vi "Puff_release3_chs.vi"() -> (5 "Plug in titles":string[](array[string]), 7 "Plug in values":string[](array[string]))   [LabVIEW 2010]
uses:
  Controls/Post_Process.ctl
  Globals/Plug_in_data_global.vi
  Globals/Meas_global.vi
  Globals/Constants_global.vi
  Globals/Dynamic_call_global.ph.vi
  <vilib>/Analysis/NI_AALPro.lvlib
panel:
  in  "Per Block Mode":T1(ring)
  in  "Averaging Samples":i32=1 min=1
  out "Valve to monitor delay (s)":dbl format="%.2f"
  out "Monitor trigger Index":dbl format="%.2f"
  out "Valve Trigger Index":dbl format="%.2f"
  out "Monitor FID":cluster{dbl, dbl, dbl[]}(graph)
  out "delay":dbl format="%.2f"
  out "Pulse Width":dbl format="%.2f"
  out "falltime":dbl format="%.2f"
  out "top":dbl format="%.2f"
  out "risetime":dbl format="%.2f"
  in  "Save Time pdf?":bool
  out "Pdf":cluster{"Axis":dbl[], dbl[]}(graph)
  in  "Histogram Time":dbl format="%.2f"
  out "Current Block No":i32
  in  "Save averaged traces?":bool
  in  "Pause Mode":T2(ring)
  in  "OK":bool
  out "No of Valid Blocks":dbl
  out "Valve Trace":dbl[](graph)
  out "FFID Trace":cluster{dbl, dbl, dbl[]}(graph)
  out "Source On":i32
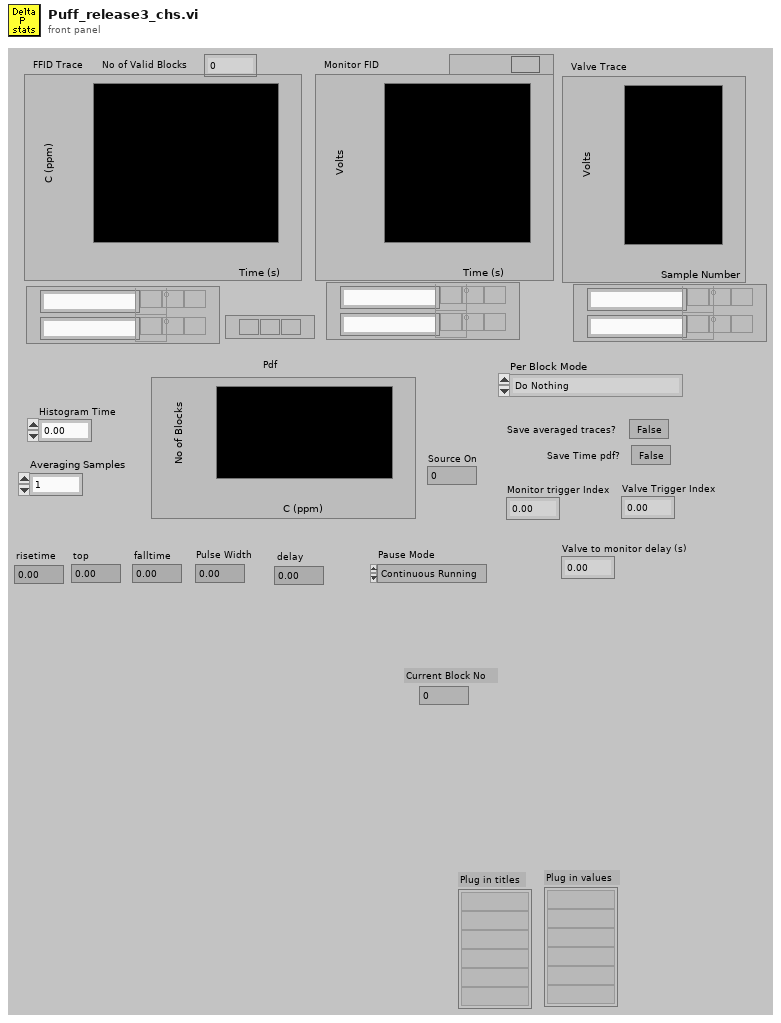
[diagram p1: front panel]
types:
  T1 = enum16{"Do Nothing", "Save Block Time Traces", "Save Jpeg plots"}
  T2 = enum16{"Continuous Running", "After Each  Block"}
  T3 = typedef "Post_Process.ctl" = enum16{"Take New Data", "Post Process Raw Data File"}
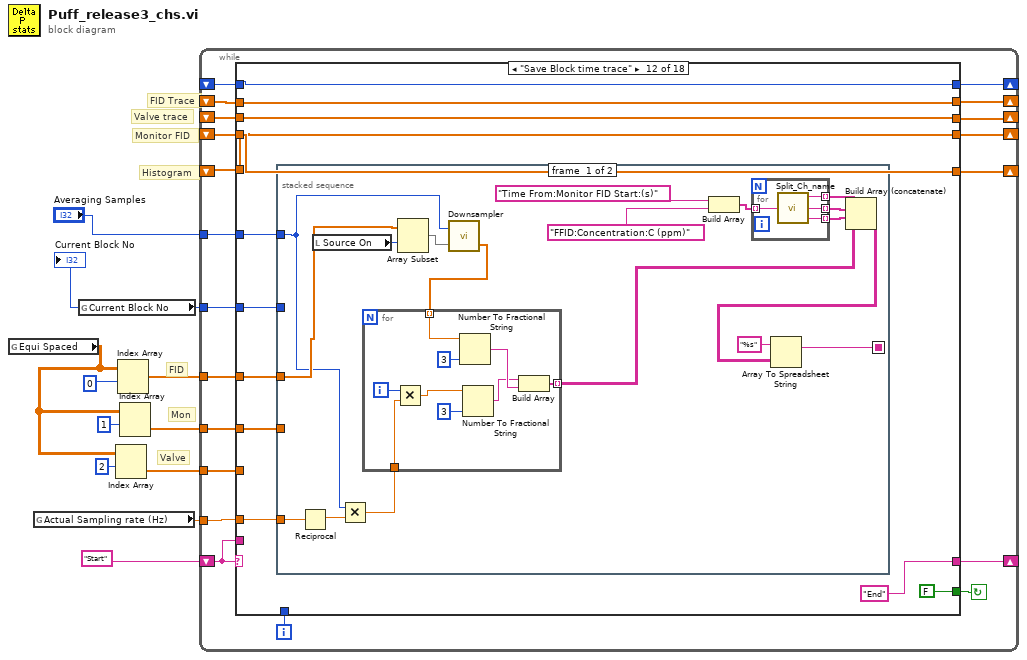
[diagram p0: block diagram]
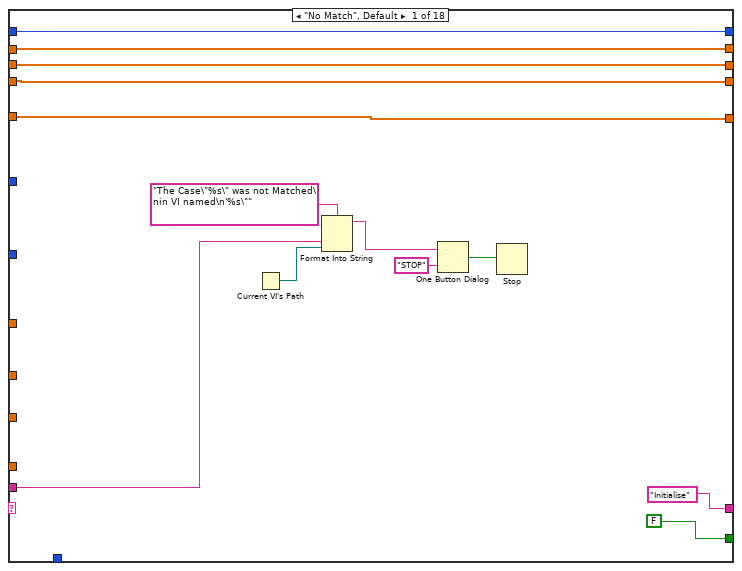
[diagram p2: hidden frame]
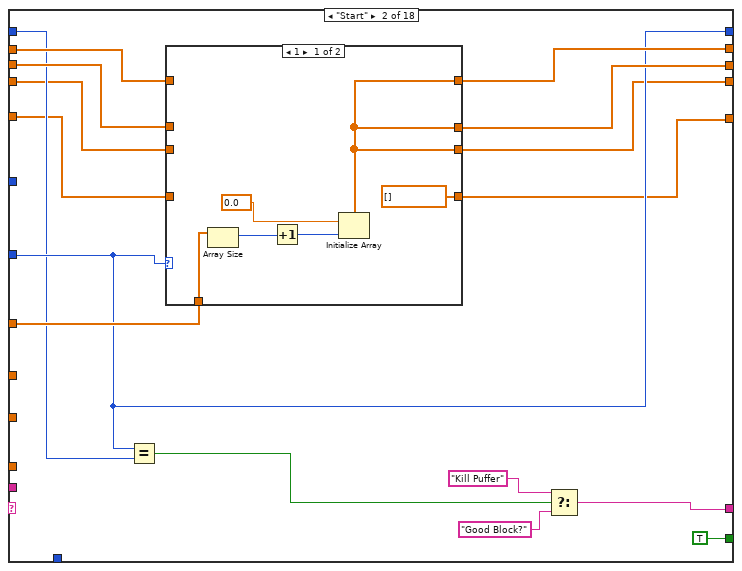
[diagram p3: hidden frame]
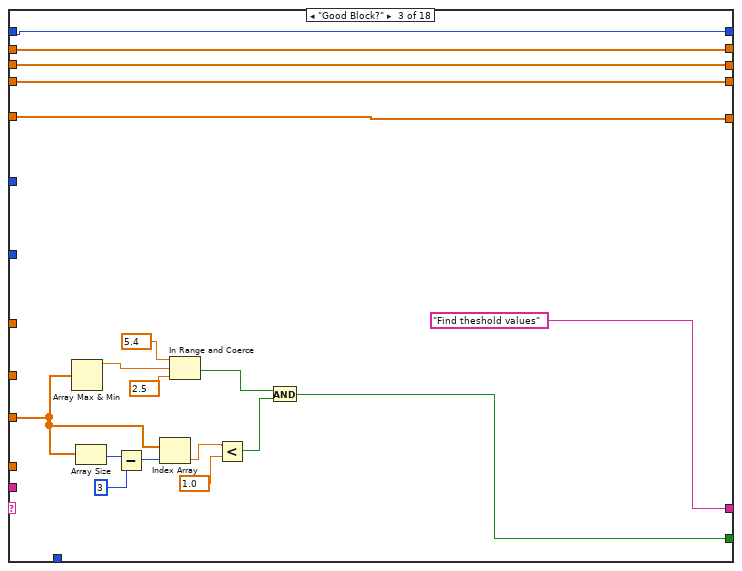
[diagram p5: hidden frame]
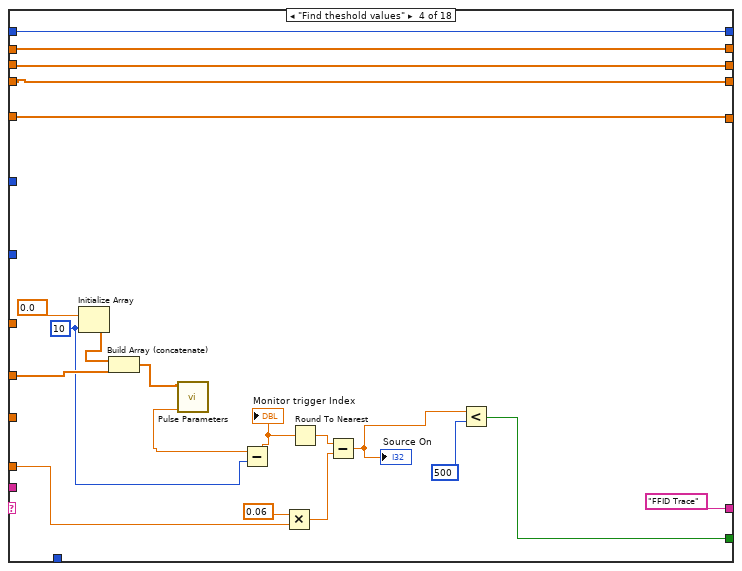
[diagram p6: hidden frame]
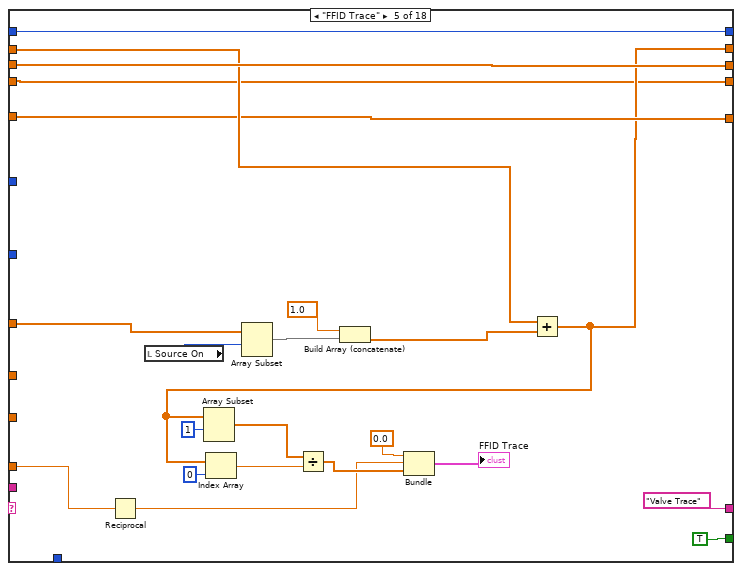
[diagram p7: hidden frame]
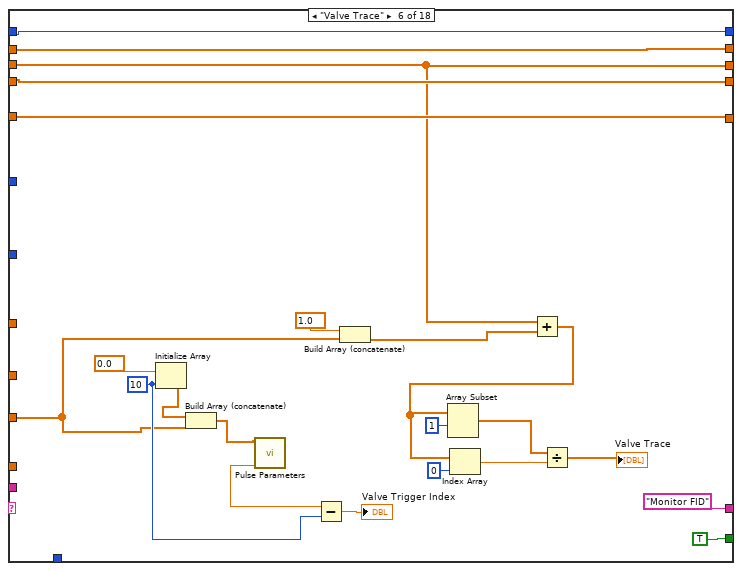
[diagram p8: hidden frame]
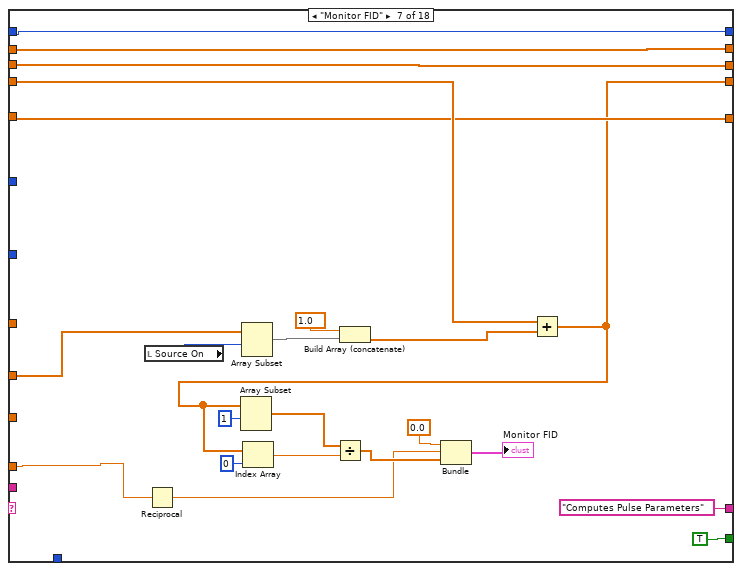
[diagram p9: hidden frame]
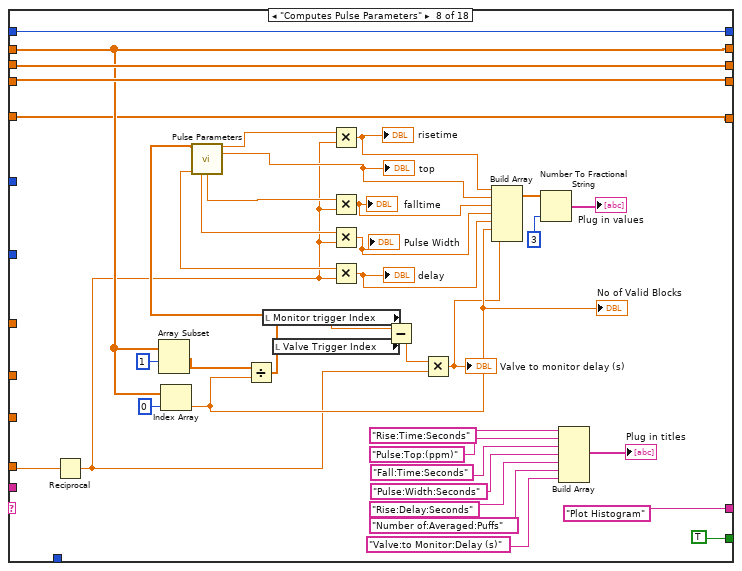
[diagram p10: hidden frame]
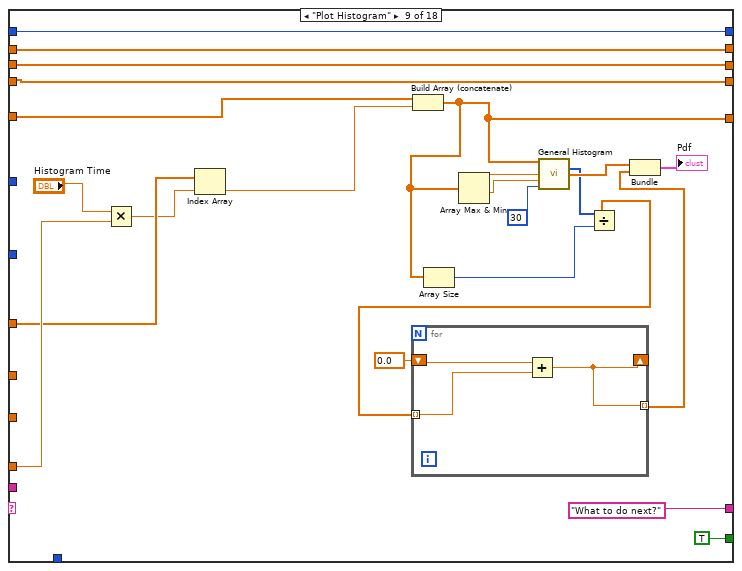
[diagram p11: hidden frame]
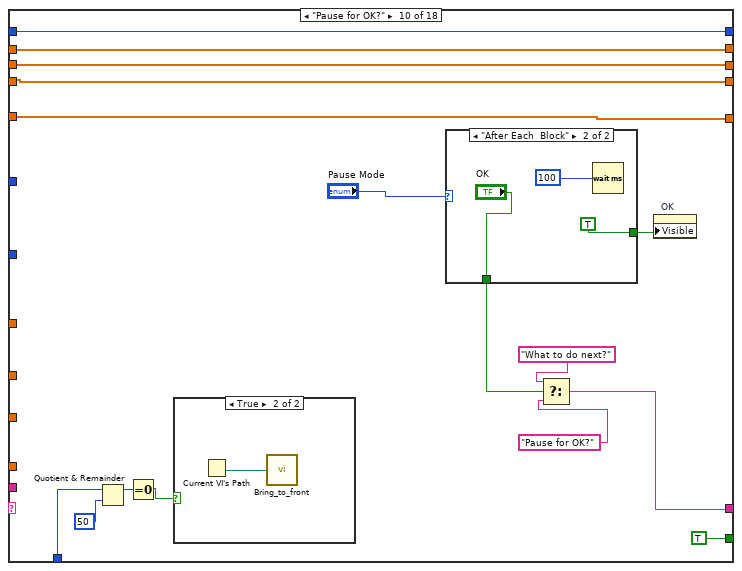
[diagram p12: hidden frame]
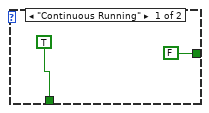
[diagram p14: hidden frame]
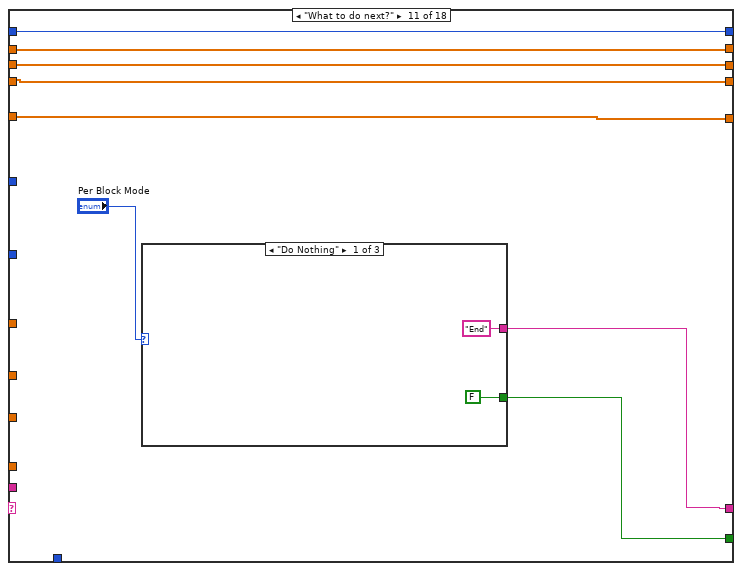
[diagram p15: hidden frame]
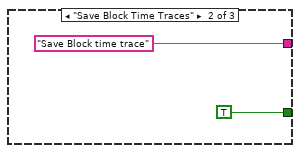
[diagram p16: hidden frame]
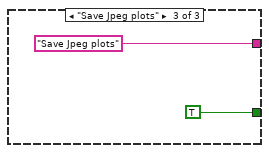
[diagram p17: hidden frame]
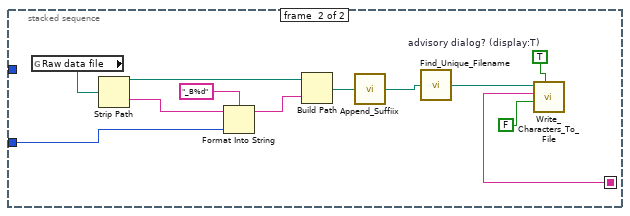
[diagram p18: hidden frame]
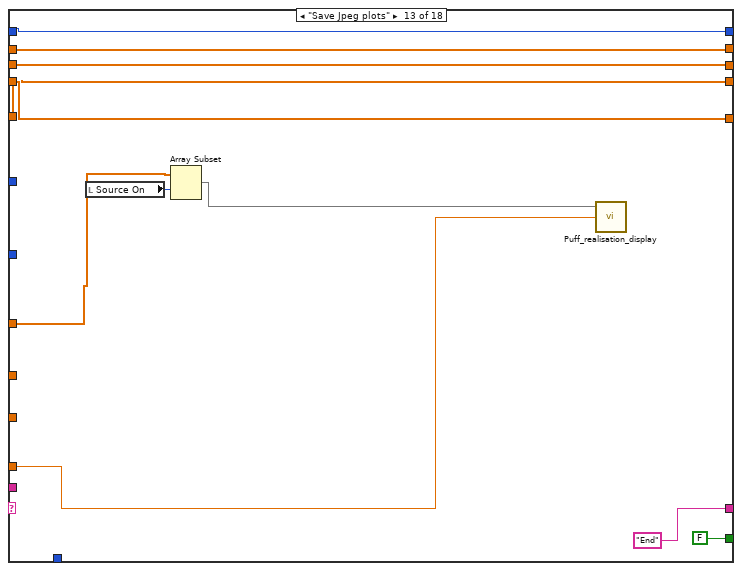
[diagram p19: hidden frame]
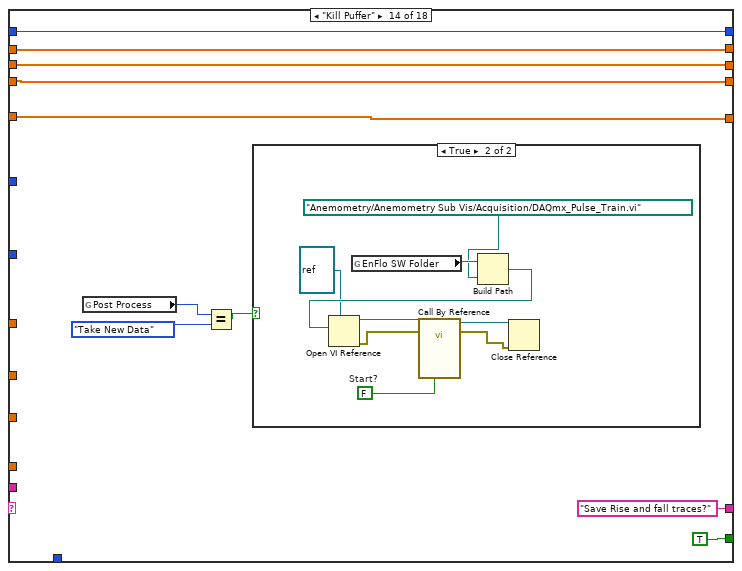
[diagram p20: hidden frame]
diagram:
  # "Valve"
  # "Mon"
  # "FID"
  # "Histogram"
  # "Monitor FID"
  # "Valve trace"
  # "FID Trace"
  n1 = global read "Plug_in_data_global.vi" "Equi Spaced"() -> (w4:dbl[][])
  n2 = global read "Meas_global.vi" "Actual Sampling rate (Hz)"() -> (w8:dbl)
  n3 = global read "Meas_global.vi" "Current Block No"() -> (w7:i32)
  "Current Block No" <- w7
  n4 = Index Array(array=w4, index (row)=2) -> (element=w3:dbl[])  [unwired: 1 in]
  n5 = Index Array(array=w4, index (row)=0) -> (element=w9:dbl[])  [unwired: 1 in]
  n6 = Index Array(array=w4, index (row)=1) -> (element=w10:dbl[])  [unwired: 1 in]
  n7 = while {
    shift-left: "Start" -> [w29]
    shift-right: [w30] -> _
    shift-right: [w28] -> _
    shift-left: _ -> [w25]
    shift-right: [w27] -> _
    shift-left: _ -> [w26]
    tunnel: w10 -> [w24]
    tunnel: w9 -> [w23]
    tunnel: w8 -> [w22]
    tunnel: w7 -> [w21]
    shift-right: [w18] -> _
    shift-left: _ -> [w19]
    shift-right: [w16] -> _
    shift-left: _ -> [w17]
    shift-right: [w14] -> _
    shift-left: _ -> [w13]
    tunnel: w3 -> [w15]
    tunnel: "Averaging Samples" -> [w12]
    i -> [w20]
    stop <- w31 continue-if-true
    n8 = case shown="\"Save Block time trace\"" w29 {
      tunnel: [FALSE TRUE ("Processing last block?") w78 w104 TRUE ("Processing last block?") TRUE ("Processing last block?") TRUE ("Processing last block?") TRUE ("Processing last block?") TRUE ("Processing last block?") TRUE ("Processing last block?") w261 FALSE ("Processing last block?") FALSE ("Processing last block?") TRUE ("Processing last block?") w360 TRUE ("Processing last block?") "Save Time pdf?" FALSE ("Processing last block?")] -> w31
      tunnel: ["Initialise" w50 "Find theshold values" "FFID Trace" "Valve Trace" "Monitor FID" "Computes Pulse Parameters" "Plot Histogram" ("f") "What to do next?" ("f") w241 w262 "End" "End" "Save Rise and fall traces?" w363 "Save Time pdf?" "Save Time pdf" "End"] -> w30
      tunnel: w29 -> [w39 _ _ _ _ _ _ _ _ _ _ _ _ _ _ _ _ _]
      tunnel: [w36 w59 w88 w107 w115 w149 w169 w182 w235 w254 w268 w286 w340 w350 w369 w376 w445 w455] -> w28
      tunnel: [w35 w57 w87 w106 w128 w131 w166 w210 w234 w253 w267 w285 w339 w349 w368 w375 w444 w454] -> w27
      tunnel: w26 -> [w35 w56 w87 w106 w128 w131 w166 w210 w234 w253 w267 w285 w339 w349 w368 w375 w444 w454]
      tunnel: w25 -> [w36 w58 w88 w107 w126 w149 w169 w182 w235 w254 w268 w286 w340 w350 w369 w376 w445 w455]
      tunnel: w24 -> [_ _ _ w100 _ _ w153 _ _ _ _ w282 _ _ _ _ _ w451]
      tunnel: w23 -> [_ w55 _ _ w127 _ _ _ w230 _ _ w281 w333 _ _ _ _ w450]
      tunnel: w22 -> [_ _ _ w94 w112 _ w154 w208 w231 _ _ w275 w330 _ _ _ _ _]
      tunnel: w21 -> [_ w54 _ _ _ _ _ _ _ _ _ w280 _ _ _ _ _ w449]
      tunnel: w20 -> [_ _ _ _ _ _ _ _ _ w251 _ _ _ _ _ _ _ _]
      tunnel: w19 -> [w34 w53 w79 w103 w121 w148 w168 w206 w233 w247 w266 w279 w336 w346 _ w372 _ w448]
      tunnel: [w34 w54 w79 w103 w121 w148 w168 w206 w233 w247 w266 w279 w336 w346 0 w372 0 w448] -> w18
      tunnel: w17 -> [w33 w47 w77 w96 w120 w141 w164 w181 w227 w246 w265 w278 w335 w342 w361 w371 w440 w446]
      tunnel: [w33 w48 w77 w96 w120 w141 w164 w181 w219 w246 w265 w278 w335 w342 w361 w371 w440 w446] -> w16
      tunnel: w15 -> [_ _ w73 _ _ w134 _ _ _ _ _ _ _ _ _ _ _ _]
      tunnel: [w32 w46 w74 w97 w109 w142 w155 w186 w216 w245 w264 w277 w334 w341 w362 w370 w439 w447] -> w14
      tunnel: w13 -> [w32 w45 w74 w97 w109 w142 w165 w186 w216 w245 w264 w277 w334 w341 w362 w370 w439 w447]
      tunnel: w12 -> [_ _ _ _ _ _ _ _ _ _ _ w276 _ _ _ _ _ _]
      frame "No Match", Default {
        n9 = Current VI's Path() -> (path=w38:path)
        n10 = Format Into String(format string="The Case\"%s\" was not Matched\nin VI named\n'%s\"" ("Format String"), w39, w38) -> (resulting string=w42:string)  [unwired: 2 in, 1 out]
        n11 = One Button Dialog(message=w42, button name ("OK")="STOP") -> (true=w40:bool)
        n12 = Stop(stop? (T)=w40) -> ()
      }
      frame "Start" {
        n13 = Equal?(x=w54, y=w53) -> (x = y?=w52:bool)
        n14 = case shown="1" w54 {
          tunnel: [w62 w70] -> w59
          tunnel: w58 -> [_ w70]
          tunnel: [w62 w69] -> w57
          tunnel: w56 -> [_ w69]
          tunnel: w55 -> [w66 _]
          tunnel: [dbl[] [] w68] -> w48
          tunnel: w47 -> [_ w68]
          tunnel: [w62 w67] -> w46
          tunnel: w45 -> [_ w67]
          frame 1 {
            n15 = Array Size(array=w66) -> (size(s)=w65:i32)
            n16 = Increment(x=w65) -> (x+1=w61:i32)
            n17 = Initialize Array(0.0 ("element"), w61) -> (w62:dbl[])
          }
          frame 2, Default {
          }
        }
        n18 = Select(t="Kill Puffer", s=w52, f="Good Block?") -> (s? t:f=w50:string)
      }
      frame "Good Block?" {
        n19 = Array Max & Min(array=w73) -> (max value=w76:dbl)  [unwired: 3 out]
        n20 = Array Size(array=w73) -> (size(s)=w72:i32)
        n21 = Subtract(x=w72, y=3) -> (x-y=w84:i32)
        n22 = Index Array(array=w73, index=w84) -> (element=w83:dbl)
        n23 = In Range and Coerce(upper limit=5.4, x=w76, lower limit=2.5 ("y")) -> (In Range?=w80:bool)  [unwired: 1 out]
        n24 = Less?(x=w83, y=1.0) -> (x < y?=w81:bool)
        n25 = And(x=w80, y=w81) -> (x .and. y?=w78:bool)
      }
      frame "Find theshold values" {
        w98 = 10 ("dimension size")
        n26 = Initialize Array(0.0, w98) -> (w99:dbl[])
        n27 = Build Array (concatenate)(w99, w100) -> (w101:dbl[])
        n28 = call <vilib>:"Pulse Parameters.vi"("X"=w101) -> ("delay"=w93:dbl)  [unwired: 14 out]
        n29 = Subtract(x=w93, y=w98) -> (x-y=w92:dbl)
        "Monitor trigger Index" <- w92
        n30 = Multiply(x=0.06 ("y"), y=w94) -> (x*y=w90:dbl)
        n31 = Round To Nearest(number=w92) -> (nearest integer value=w91:dbl)
        n32 = Subtract(x=w91, y=w90) -> (x-y=w89:dbl)
        "Source On" <- w89
        n33 = Less?(x=w89, y=500) -> (x < y?=w104:bool)
      }
      frame "FFID Trace" {
        n34 = Reciprocal(x=w112) -> (1/x=w111:dbl)
        n35 = local read "Source On"() -> (w123:i32)
        n36 = Array Subset(array=w127, index=w123) -> (w122:dbl[])  [unwired: 1 in]
        n37 = Build Array (concatenate)(1.0, w122) -> (w124:dbl[])
        n38 = Add(x=w126, y=w124) -> (x+y=w115:dbl[])
        n39 = Array Subset(array=w115, index=1) -> (w114:dbl[])  [unwired: 1 in]
        n40 = Index Array(array=w115, index=0) -> (element=w113:dbl)
        n41 = Divide(x=w114, y=w113) -> (x/y=w119:dbl[])
        n42 = Bundle(0.0, w111, w119) -> (→"FFID Trace":cluster{dbl, dbl, dbl[]})  [unwired: 1 out]
      }
      frame "Valve Trace" {
        w135 = 10 ("dimension size")
        n43 = Initialize Array(0.0, w135) -> (w136:dbl[])
        n44 = Build Array (concatenate)(w136, w134) -> (w137:dbl[])
        n45 = call <vilib>:"Pulse Parameters.vi"("X"=w137) -> ("delay"=w132:dbl)  [unwired: 14 out]
        n46 = Subtract(x=w132, y=w135) -> (x-y=→"Valve Trigger Index":dbl)
        n47 = Build Array (concatenate)(1.0, w134) -> (w150:dbl[])
        n48 = Add(x=w131, y=w150) -> (x+y=w139:dbl[])
        n49 = Array Subset(array=w139, index=1) -> (w144:dbl[])  [unwired: 1 in]
        n50 = Index Array(array=w139, index=0) -> (element=w143:dbl)
        n51 = Divide(x=w144, y=w143) -> (x/y=→"Valve Trace":dbl[])
      }
      frame "Monitor FID" {
        n52 = local read "Source On"() -> (w171:i32)
        n53 = Reciprocal(x=w154) -> (1/x=w157:dbl)
        n54 = Array Subset(array=w153, index=w171) -> (w170:dbl[])  [unwired: 1 in]
        n55 = Build Array (concatenate)(1.0, w170) -> (w172:dbl[])
        n56 = Add(x=w165, y=w172) -> (x+y=w155:dbl[])
        n57 = Array Subset(array=w155, index=1) -> (w159:dbl[])  [unwired: 1 in]
        n58 = Index Array(array=w155, index=0) -> (element=w158:dbl)
        n59 = Divide(x=w159, y=w158) -> (x/y=w163:dbl[])
        n60 = Bundle(0.0, w157, w163) -> (→"Monitor FID":cluster{dbl, dbl, dbl[]})  [unwired: 1 out]
      }
      frame "Computes Pulse Parameters" {
        n61 = Reciprocal(x=w208) -> (1/x=w177:dbl)
        n62 = Array Subset(array=w182, index=1) -> (w185:dbl[])  [unwired: 1 in]
        n63 = Index Array(array=w182, index=0) -> (element=w184:dbl)
        "No of Valid Blocks" <- w184
        n64 = Divide(x=w185, y=w184) -> (x/y=w183:dbl[])
        n65 = call <vilib>:"Pulse Parameters.vi"("X"=w183) -> ("risetime"=w205:dbl, "top"=w191:dbl, "delay"=w202:dbl, "duration"=w203:dbl, "falltime"=w204:dbl)  [unwired: 10 out]
        "top" <- w191
        n66 = local read "Monitor trigger Index"() -> (w179:dbl)
        n67 = local read "Valve Trigger Index"() -> (w180:dbl)
        n68 = Multiply(x=w205, y=w177) -> (x*y=w190:dbl)
        "risetime" <- w190
        n69 = Multiply(x=w204, y=w177) -> (x*y=w189:dbl)
        "falltime" <- w189
        n70 = Multiply(x=w203, y=w177) -> (x*y=w188:dbl)
        "Pulse Width" <- w188
        n71 = Multiply(x=w202, y=w177) -> (x*y=w187:dbl)
        "delay" <- w187
        n72 = Subtract(x=w179, y=w180) -> (x-y=w178:dbl)
        n73 = Multiply(x=w178, y=w177) -> (x*y=w176:dbl)
        "Valve to monitor delay (s)" <- w176
        n74 = Build Array(w190, w191, w189, w188, w187, w184, w176) -> (w201:dbl[])
        n75 = Number To Fractional String(number=w201, precision (6)=i16 3) -> (F-format string=→"Plug in values":string[])  [unwired: 2 out]
        n76 = Build Array("Rise:Time:Seconds", "Pulse:Top:(ppm)", "Fall:Time:Seconds", "Pulse:Width:Seconds", "Rise:Delay:Seconds", "Number of:Averaged:Puffs", "Valve:to Monitor:Delay (s)") -> (→"Plug in titles":string[])
      }
      frame "Plot Histogram" {
        n77 = Multiply(x="Histogram Time", y=w231) -> (x*y=w229:dbl)
        n78 = Index Array(array=w230, index=w229) -> (element=w228:dbl)
        n79 = Build Array (concatenate)(w227, w228) -> (w219:dbl[])
        n80 = Array Size(array=w219) -> (size(s)=w217:i32)
        n81 = Array Max & Min(array=w219) -> (max value=w226:dbl, min value=w225:dbl)  [unwired: 2 out]
        n82 = call <vilib>:"General Histogram.vi"("X"=w219, "max"=w226, "min"=w225, "# bins"=30) -> ("Histogram"=w218:i32[], "Axis"=w223:dbl[])  [unwired: 2 in, 8 out]
        n83 = Divide(x=w218, y=w217) -> (x/y=w213:dbl[])
        n84 = for {
          shift-right: [w236] -> _
          shift-left: 0.0 -> [w238]
          tunnel: w213 -> [w237] mode=indexing
          tunnel: [w236] -> w214 mode=indexing
          n85 = Add(x=w238, y=w237) -> (x+y=w236:dbl)
        }
        n86 = Bundle("Axis"=w223, w214) -> (→"Pdf":cluster{"Axis":dbl[], dbl[]})  [unwired: 1 out]
      }
      frame "Pause for OK?" {
        n87 = Quotient & Remainder(x=w251, y=50) -> (x-y*floor(x/y)=w249:i32)  [unwired: 1 out]
        n88 = Equal To 0?(x=w249) -> (x = 0?=w248:bool)
        n89 = case shown="True" w248 {
          frame False {
          }
          frame True {
            n90 = Current VI's Path() -> (path=w255:path)
            n91 = call "Bring_to_front.vi"("path"=w255) -> ()
          }
        }
        n92 = case shown="\"After Each  Block\"" "Pause Mode" {
          tunnel: [TRUE "OK"] -> w242
          tunnel: [FALSE TRUE] -> w252
          frame "Continuous Running" {
          }
          frame "After Each  Block" {
            n93 = Wait (ms)(milliseconds to wait=u32 100 ("f")) -> ()  [unwired: 1 out]
          }
        }
        n94 = Select(t="What to do next?" ("f"), s=w242, f="Pause for OK?") -> (s? t:f=w241:string)
        n95 = property on="OK" class="Bool"("Visible"=w252) -> ()  [unwired: 2 in, 2 out]
      }
      frame "What to do next?" {
        n96 = case shown="\"Do Nothing\"" "Per Block Mode" {
          tunnel: ["End" ("t") "Save Block time trace" ("t") "Save Jpeg plots" ("t")] -> w262
          tunnel: [FALSE TRUE TRUE] -> w261
          frame "Do Nothing" {
          }
          frame "Save Block Time Traces" {
          }
          frame "Save Jpeg plots" {
          }
        }
      }
      frame "Save Block time trace" {
        n97 = stacked-sequence {
          seq-local: [w300 _] -> [_ w326]
          tunnel: w282 -> [_ _]
          tunnel: w281 -> [w297 _]
          tunnel: w280 -> [_ w323]
          tunnel: w276 -> [w292 _]
          tunnel: w275 -> [w294 _]
          frame #0 {
            n98 = Reciprocal(x=w294) -> (1/x=w293:dbl)
            n99 = local read "Source On"() -> (w298:i32)
            n100 = Multiply(x=w292, y=w293) -> (x*y=w291:dbl)
            n101 = Array Subset(array=w297, index=w298) -> (w296:dbl[])  [unwired: 1 in]
            n102 = call "Downsampler.vi"("Input Array"=w296, "Averaging samples"=w292) -> ("Downsampled Array"=w295:dbl[])  [unwired: 1 out]
            n103 = for {
              tunnel: [w315] -> w299 mode=indexing
              tunnel: w295 -> [w312] mode=indexing
              tunnel: w291 -> [w311]
              i -> [w310]
              n104 = Multiply(x=w310, y=w311) -> (x*y=w309:dbl)
              n105 = Number To Fractional String(number=w312, precision (6)=i16 3) -> (F-format string=w314:string)  [unwired: 2 out]
              n106 = Number To Fractional String(number=w309, precision (6)=i16 3) -> (F-format string=w313:string)  [unwired: 2 out]
              n107 = Build Array(w313, w314) -> (w315:string[])
            }
            n108 = Build Array("Time From:Monitor FID Start:(s)", "FFID:Concentration:C (ppm)") -> (w290:string[])
            n109 = for {
              tunnel: w290 -> [w308] mode=indexing
              tunnel: [w307] -> w289 mode=indexing
              tunnel: [w306] -> w288 mode=indexing
              tunnel: [w305] -> w287 mode=indexing
              n110 = call "Split_Ch_name.vi"("Ch name"=w308) -> ("Top level"=w307:string, "Middle"=w306:string, "Low level"=w305:string)
            }
            n111 = Build Array (concatenate)(w289, w288, w287, w299) -> (w302:string[][])
            n112 = Array To Spreadsheet String(array=w302, 3:"%s" ("format string")) -> (spreadsheet string=w300:string)  [unwired: 1 out]
          }
          frame #1 {
            w328 = TRUE  # advisory dialog? (display:T)
            n113 = global read "Meas_global.vi" "Raw data file"() -> (w329:path)
            n114 = Strip Path(path=w329) -> (stripped path=w325:path, name=w324:string)
            n115 = Format Into String(format string="_B%d", initial string=w324, w323) -> (resulting string=w321:string)  [unwired: 1 in, 1 out]
            n116 = Build Path(base path=w325, name or relative path=w321) -> (appended path=w320:path)
            n117 = call "Append_Suffiix.vi"("Results file"=w320) -> ("appended path"=w319:path)
            n118 = call "Find_Unique_Filename.vi"("Path In"=w319) -> ("Unique Path Out"=w318:path)  [unwired: 1 in, 1 out]
            n119 = call "Write_Characters_To_File.vi"("file path (dialog if empty)"=w318, "advisory dialog? (display:T)"=w328, "character string"=w326, "append to file? (new file:F)"=FALSE) -> ()  [unwired: 1 in, 4 out]
          }
        }
      }
      frame "Save Jpeg plots" {
        n120 = local read "Source On"() -> (w332:i32)
        n121 = Array Subset(array=w333, index=w332) -> (w331:dbl[])  [unwired: 1 in]
        n122 = call "Puff_realisation_display.vi"("Actual Sampling rate (Hz)"=w330, "Input Array"=w331) -> ()  [unwired: 2 out]
      }
      frame "Kill Puffer" {
        n123 = global read "Meas_global.vi" "Post Process"() -> (w345:T3)
        n124 = Equal?(x=w345, y=Post_Process."Take New Data" ("Post Process")) -> (x = y?=w343:bool)
        n125 = case shown="True" w343 {
          frame False {
          }
          frame True {
            w359 = FALSE  # Start?
            n126 = global read "Constants_global.vi" "EnFlo SW Folder"() -> (w358:path)
            n127 = Build Path(base path=w358, name or relative path=path "Anemometry/Anemometry Sub Vis/Acquisition/DAQmx_Pulse_Train.vi") -> (appended path=w356:path)
            n128 = Open VI Reference(type specifier VI Refnum (for type only)=refnum<vi> refnum, vi path=w356) -> (vi reference=w355:refnum<vi>, error out=w352:errorcluster)  [unwired: 1 in, 3 out]
            n129 = call-by-ref "?"(reference=w355, error in=w352, "Start?"=w359) -> (reference out=w353:refnum<vi>, error out=w351:errorcluster)  [unwired: 8 in]
            n130 = Close Reference(reference=w353, error in (no error)=w351) -> ()  [unwired: 1 out]
          }
        }
      }
      frame "Save Rise and fall traces?" {
        n131 = Select(t="Write Results file", s="Save averaged traces?", f="Save Time PDF?") -> (s? t:f=w363:string)
        n132 = global read "Meas_global.vi" "Processing last block?"() -> (w360:bool)
      }
      frame "Write Results file" {
        n133 = stacked-sequence {
          seq-local: [w385 _] -> [_ w415]
          frame #0 {
            n134 = local read "FFID Trace"() -> (w395:cluster{dbl, dbl, dbl[]})
            n135 = local read "Monitor FID"() -> (w384:cluster{dbl, dbl, dbl[]})
            n136 = Unbundle(w395) -> (w393:dbl, w394:dbl, w392:dbl[])
            n137 = Unbundle(w384) -> (w383:dbl[])  [unwired: 2 out]
            n138 = for {
              tunnel: w394 -> [w406]
              tunnel: w393 -> [w405]
              tunnel: w392 -> [w400] mode=indexing
              tunnel: [w403] -> w390 mode=indexing
              tunnel: w383 -> [w401] mode=indexing
              i -> [w407]
              n139 = Multiply(x=w406, y=w407) -> (x*y=w404:dbl)
              n140 = Add(x=w405, y=w404) -> (x+y=w402:dbl)
              n141 = Build Array(w402, w401, w400) -> (w403:dbl[])
            }
            n142 = Build Array("Time From:Monitor FID Start:(s)", "Monitor FID:Voltage:Trace", "FFID:Concentration:C (ppm)") -> (w380:string[])
            n143 = for {
              tunnel: w380 -> [w399] mode=indexing
              tunnel: [w398] -> w379 mode=indexing
              tunnel: [w397] -> w378 mode=indexing
              tunnel: [w396] -> w377 mode=indexing
              n144 = call "Split_Ch_name.vi"("Ch name"=w399) -> ("Top level"=w398:string, "Middle"=w397:string, "Low level"=w396:string)
            }
            n145 = Number To Fractional String(number=w390, precision (6)=i16 3) -> (F-format string=w389:string[][])  [unwired: 2 out]
            n146 = Build Array (concatenate)(w379, w378, w377, w389) -> (w387:string[][])
            n147 = Array To Spreadsheet String(array=w387, 3:"%s" ("format string")) -> (spreadsheet string=w385:string)  [unwired: 1 out]
          }
          frame #1 {
            w430 = TRUE  # advisory dialog? (display:T)
            n148 = global read "Dynamic_call_global.ph.vi" "Plug in titles"() -> (w427:string[])
            n149 = global read "Dynamic_call_global.ph.vi" "Plug in values"() -> (w423:string[])
            n150 = global read "Meas_global.vi" "Raw data file"() -> (w434:path)
            n151 = Strip Path(path=w434) -> (stripped path=w428:path, name=w413:string)
            n152 = String Subset(string=w413, offset (0)=0, length (rest)=28 ("length (rest)")) -> (substring=w410:string)
            n153 = for {
              tunnel: w427 -> [w438] mode=indexing
              tunnel: [w437] -> w426 mode=indexing
              tunnel: [w436] -> w425 mode=indexing
              tunnel: [w435] -> w424 mode=indexing
              n154 = call "Split_Ch_name.vi"("Ch name"=w438) -> ("Top level"=w437:string, "Middle"=w436:string, "Low level"=w435:string)
            }
            n155 = Concatenate Strings(w410, "_Av" ("string")) -> (w433:string)
            n156 = Initialize Array("", 15) -> (w420:string[])
            n157 = Build Path(base path=w428, name or relative path=w433) -> (appended path=w409:path)
            n158 = call "Append_Suffiix.vi"("Results file"=w409) -> ("appended path"=w408:path)
            n159 = call "Asterisk_header.vi"("Channel names"=w420) -> ("Header string"=w416:string)
            n160 = call "Find_Unique_Filename.vi"("Path In"=w408) -> ("Unique Path Out"=w431:path)  [unwired: 1 in, 1 out]
            n161 = Build Array(w426, w425, w424, w423) -> (w421:string[][])
            n162 = Array To Spreadsheet String(array=w421, 3:"%s" ("format string")) -> (spreadsheet string=w417:string)  [unwired: 1 out]
            n163 = Concatenate Strings(w417, w416, w415) -> (w414:string)
            n164 = call "Write_Characters_To_File.vi"("file path (dialog if empty)"=w431, "advisory dialog? (display:T)"=w430, "character string"=w414, "append to file? (new file:F)"=FALSE) -> ()  [unwired: 1 in, 4 out]
          }
        }
      }
      frame "Save Time pdf?" {
      }
      frame "Save Time pdf" {
        n165 = stacked-sequence {
          seq-local: [w464 _] -> [_ w485]
          tunnel: w451 -> [_ _]
          tunnel: w450 -> [_ _]
          tunnel: w449 -> [_ _]
          frame #0 {
            n166 = local read "Pdf"() -> (w462:cluster{"Axis":dbl[], dbl[]})
            n167 = Unbundle(w462) -> ("Axis"=w461:dbl[], w460:dbl[])
            n168 = for {
              tunnel: w460 -> [w478] mode=indexing
              tunnel: w461 -> [w477] mode=indexing
              tunnel: [w476] -> w463 mode=indexing
              n169 = Number To Fractional String(number=w478, precision (6)=i16 3) -> (F-format string=w474:string)  [unwired: 2 out]
              n170 = Number To Fractional String(number=w477, precision (6)=i16 3) -> (F-format string=w475:string)  [unwired: 2 out]
              n171 = Build Array(w475, w474) -> (w476:string[])
            }
            n172 = Build Array("FFID:Concentration:C (ppm)", "Pdf:Bin:Frequency") -> (w459:string[])
            n173 = for {
              tunnel: w459 -> [w472] mode=indexing
              tunnel: [w471] -> w458 mode=indexing
              tunnel: [w470] -> w457 mode=indexing
              tunnel: [w469] -> w456 mode=indexing
              n174 = call "Split_Ch_name.vi"("Ch name"=w472) -> ("Top level"=w471:string, "Middle"=w470:string, "Low level"=w469:string)
            }
            n175 = Build Array (concatenate)(w458, w457, w456, w463) -> (w466:string[][])
            n176 = Array To Spreadsheet String(array=w466, 3:"%s" ("format string")) -> (spreadsheet string=w464:string)  [unwired: 1 out]
          }
          frame #1 {
            w503 = TRUE  # advisory dialog? (display:T)
            n177 = global read "Dynamic_call_global.ph.vi" "Plug in titles"() -> (w497:string[])
            n178 = global read "Dynamic_call_global.ph.vi" "Plug in values"() -> (w493:string[])
            n179 = global read "Meas_global.vi" "Raw data file"() -> (w506:path)
            n180 = local read "Histogram Time"() -> (w498:dbl)
            n181 = Strip Path(path=w506) -> (stripped path=w501:path, name=w481:string)
            n182 = String Subset(string=w481, offset (0)=0, length (rest)=20 ("length (rest)")) -> (substring=w480:string)
            n183 = for {
              tunnel: w497 -> [w510] mode=indexing
              tunnel: [w509] -> w496 mode=indexing
              tunnel: [w508] -> w495 mode=indexing
              tunnel: [w507] -> w494 mode=indexing
              n184 = call "Split_Ch_name.vi"("Ch name"=w510) -> ("Top level"=w509:string, "Middle"=w508:string, "Low level"=w507:string)
            }
            n185 = Format Into String(format string="_T=%.2f", initial string=w480, w498) -> (resulting string=w499:string)  [unwired: 1 in, 1 out]
            n186 = Initialize Array("", 15) -> (w490:string[])
            n187 = Build Path(base path=w501, name or relative path=w499) -> (appended path=w505:path)
            n188 = call "Asterisk_header.vi"("Channel names"=w490) -> ("Header string"=w486:string)
            n189 = call "Find_Unique_Filename.vi"("Path In"=w505) -> ("Unique Path Out"=w504:path)  [unwired: 1 in, 1 out]
            n190 = Build Array(w496, w495, w494, w493) -> (w491:string[][])
            n191 = Array To Spreadsheet String(array=w491, 3:"%s" ("format string")) -> (spreadsheet string=w487:string)  [unwired: 1 out]
            n192 = Concatenate Strings(w487, w486, w485) -> (w484:string)
            n193 = call "Write_Characters_To_File.vi"("file path (dialog if empty)"=w504, "advisory dialog? (display:T)"=w503, "character string"=w484, "append to file? (new file:F)"=FALSE) -> ()  [unwired: 1 in, 4 out]
          }
        }
      }
    }
  }
